vi "Run Child.vi"(8 "error in (no error)":errorcluster, 9 "Working Path":path, 10 "UI":refnum<class "UI.lvclass">, 11 "Remove in":refnum<class "Remove.lvclass">) -> (0 "error out":errorcluster, 3 "Remove out":refnum<class "Remove.lvclass">)   [LabVIEW 2020, in "Remove.lvlib" / "Remove.lvclass"]
uses:
  Remove.lvclass
  build/ppl/neg-pkg.lvlibp/neg-pkg/UI/UI.lvclass
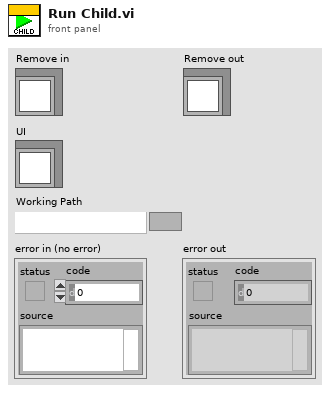
[diagram p1: front panel]
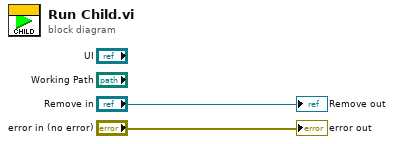
[diagram p0: block diagram]
diagram:
  "error out" <- "error in (no error)"
  "Remove out" <- "Remove in"
